vi "5.2.vi"() -> ()   [LabVIEW 2022 SP3]
panel:
  out "Addition With Filter":dynamicdata(graph) caption="Square with Uniform Noise"
  out "Addition Without Filter":dynamicdata(graph) caption="Square with Uniform Noise"
  out "Square":dynamicdata(graph) caption="Square with Uniform Noise"
  out "Sinusoid":dynamicdata(graph) caption="Square with Uniform Noise"
  # "Aditya Singh \n   2315005"
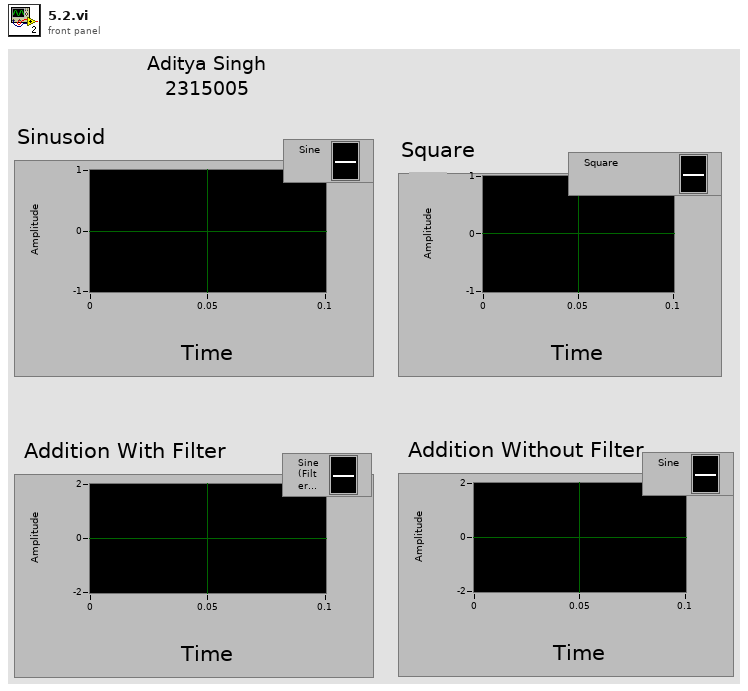
[diagram p1: front panel]
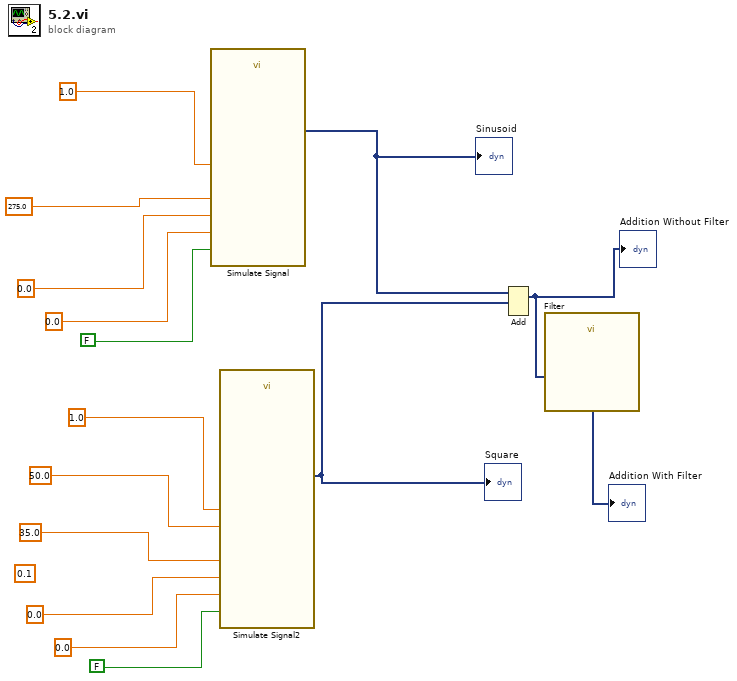
[diagram p0: block diagram]
diagram:
  (unwired) 0.1 ("Noise amplitude")
  n1 = call "Simulate Signal"("Offset"=0.0, "Reset Signal"=FALSE, "Frequency"=275.0, "Amplitude"=1.0, "Phase"=0.0) -> ("Sine"=w4:dynamicdata)  [unwired: 9 in, 1 out]
  "Sinusoid" <- w4
  n2 = call "Simulate Signal2"("Offset"=0.0, "Duty Cycle (%)"=50.0, "Reset Signal"=FALSE, "Frequency"=35.0, "Amplitude"=1.0, "Phase"=0.0) -> ("Square"=w3:dynamicdata)  [unwired: 8 in, 1 out]
  "Square" <- w3
  n3 = Add(1:w3, 2:w4) -> (0:w2:dynamicdata)  [unwired: 1 in, 1 out]
  "Addition Without Filter" <- w2
  n4 = call "Filter"("Signal"=w2) -> ("Filtered Signal"=→"Addition With Filter":dynamicdata)  [unwired: 9 in, 1 out]
